vi "Read Integer.vi"(8 "error in":errorcluster, 10 "PLC Address":string="N7:0", 11 "IP Address:":string="192.168.100.15") -> (0 "error out":errorcluster, 3 "Element:":i16)   [LabVIEW 2018]
uses:
  <vilib>/ethernetip/ethernetip.lvlib
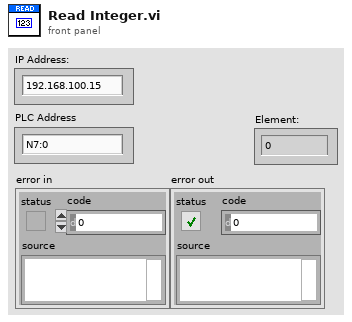
[diagram p1: front panel]
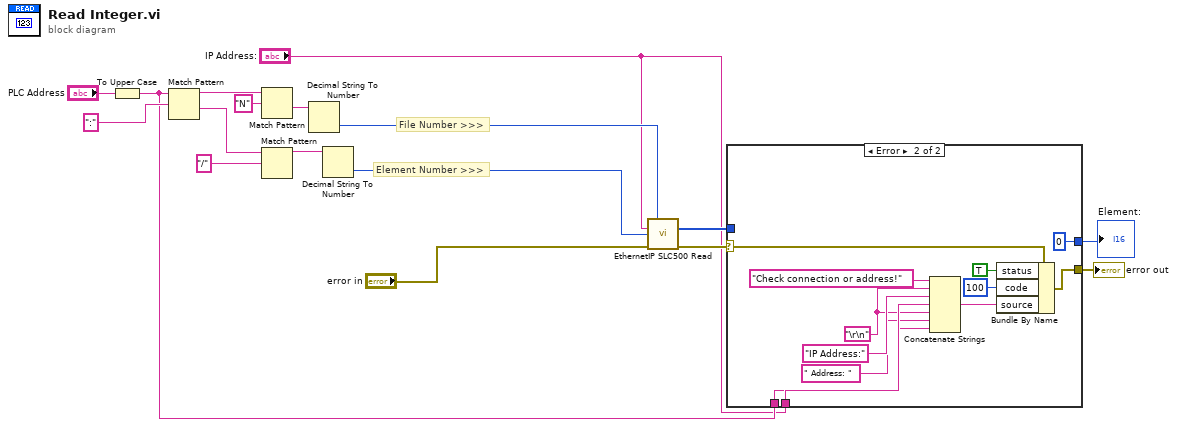
[diagram p0: block diagram]
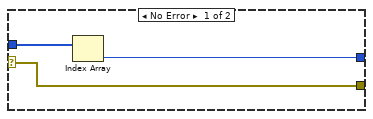
[diagram p2: hidden frame]
diagram:
  # "Element Number >>>"
  # "File Number >>>"
  n1 = To Upper Case(1:"PLC Address") -> (0:w3:string)
  n2 = Match Pattern(string=w3, regular expression=":") -> (before substring=w16:string, after substring=w11:string)  [unwired: 1 in, 2 out]
  n3 = Match Pattern(string=w16, regular expression="N") -> (after substring=w13:string)  [unwired: 1 in, 3 out]
  n4 = Match Pattern(string=w11, regular expression="/") -> (before substring=w9:string)  [unwired: 1 in, 3 out]
  n5 = Decimal String To Number(string=w13) -> (number=w12:i32)  [unwired: 2 in, 1 out]
  n6 = Decimal String To Number(string=w9) -> (number=w8:i32)  [unwired: 2 in, 1 out]
  n7 = call-poly <vilib>:"EthernetIP SLC500 Read.vi"("File Number"=w12, "Network Path"="IP Address:", "Element Number"=w8, "error in"="error in") -> ("Data"=w5:i16[], "error out"=w6:errorcluster)  [unwired: 9 in, 1 out]
  n8 = case shown="Error" w6 {
    selector: w6 -> [w19 w32]
    tunnel: w5 -> [w20 _]
    tunnel: [w19 w31] -> w4
    tunnel: w3 -> [_ w22]
    tunnel: "IP Address:" -> [_ w25]
    tunnel: [w18 i16 0] -> w1
    frame No Error {
      n9 = Index Array(array=w20) -> (element=w18:i16)  [unwired: 1 in]
    }
    frame Error {
      w24 = "\r\n"
      n10 = Concatenate Strings("Check connection or address!" ("source"), w24, "IP Address:", w25, w24, " Address: ", w22) -> (w26:string)
      n11 = Bundle By Name(cluster=w32, "status"=TRUE, "code"=100, "source"=w26) -> (w31:errorcluster)
    }
  }
  "error out" <- w4
  "Element:" <- w1
